vi "Instrument - Manual Object.vi"() -> ()   [LabVIEW 2020, in "Instrument Workspace Objects.lvlib"]
doc: "Sample numeric display item."
uses:
  Instrument Workspace Objects.lvlib
  <vilib>/NI VeriStand/Display Template Support/DisplayTemplateSupport.llb/cluster_Screen Item Settings.ctl
  <vilib>/NI VeriStand/Display Template Support/DisplayTemplateSupport.llb/cluster_Graph Scale Settings.ctl
  <vilib>/NI VeriStand/Display Template Support/DisplayTemplateSupport.llb/cluster_Graph Plot Settings.ctl
  NationalInstruments.VeriStand.SystemStorage
  Addon/Addon Shared/Types/Response Wait Type.ctl
  Workspace Shared/Types/State Variables.ctl
  <vilib>/NI VeriStand/Execution/Workspace/WorkspaceAPI.ctl
  <vilib>/NI VeriStand/Display Template Support/DisplayTemplateSupport.llb/enum_Display Template Handler Minimal To Workspace.ctl
  <vilib>/NI VeriStand/Display Template Support/DisplayTemplateSupport.llb/enum_Display Template Handler Minimal To Widget Msg.ctl
  <vilib>/NI/STM/TCP/TCP Connection Info.ctl
  <vilib>/NI/STM/SubVIs/MetaDataElement.ctl
  Workspace Shared/Types/CD Saved State.ctl
  <vilib>/NI VeriStand/Execution/Workspace/SystemStateEventRef.ctl
  <vilib>/NI VeriStand/Execution/Workspace/Target State Info.ctl
  <vilib>/NI VeriStand/Execution/Workspace/Target State.ctl
  <vilib>/NI VeriStand/Execution/Workspace/SystemStateRegEventRef.ctl
  Addon/Addon Shared/Types/Buffered RT Instrument Command.ctl
  <vilib>/NI VeriStand/Display Template Support/DisplayTemplateSupport.llb/sub_Display Template Handler Custom.vi
  Workspace Shared/Instrument Workspace Shared.lvlib
  <vilib>/NI VeriStand/Execution/Workspace/NI_VS Workspace ExecutionAPI.lvlib
  <vilib>/NI/STM/NI STM.lvlib
  APIs/Host Automation API/Instrument Host Automation API.lvlib
  Addon/Addon Shared/Instrument Addon Shared.lvlib
  NationalInstruments.VeriStand.ClientAPI
panel:
  in  "Command":string
  in  "Response?":bool
  in  "Wait Type":T1
  in  "Wait Value":dbl=100.0 format="%#_p"
  out "Timed Out?":bool
  out "Error Report":errorcluster
  out "Response":string
  in  "Send":bool
  out "Device":string
  in  "NIVS.Gateway IP Address":string
  in  "NIVS.System Definition Root":refnum<k24>
  in  "Item.Data":T2
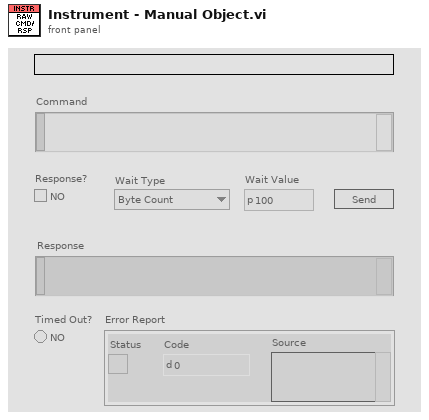
[diagram p1: front panel]
types:
  T1 = typedef "Instrument Addon Shared.lvlib/Response Wait Type.ctl" = enum16{"Byte Count", "Wait sec"}
  T2 = typedef "cluster_Screen Item Settings.ctl" = cluster{"Template VI":string, "Position X":i32, "Position Y":i32, "Custom":string, "Show Title Bar":bool, "ID":i32, "Always On Top":bool, "Allow Resize":bool, "Allow Minimize":bool, "Allow Close":bool, "Size to Screen":bool, "Screen.ID":i32, "State":enum16{"Normal", "New"}, "Title":string, "Window Bounds":cluster{"[0]":i16, "[1]":i16, "[2]":i16, "[3]":i16}, "Channel Ref":u64, "Unit":string, "Default Units?":bool, "Flash Limit?":bool, "Color 1":u32, "Color 2":u32, "Color 3":u32, "Color 4":u32, "Bck Color":u32, "Fore Color":u32, "Limit 1":dbl, "Limit 2":dbl, "Limit 3":dbl, "Limit 4":dbl, "Limit Mode 1":i32, "Limit Mode 2":i32, "Limit Mode 3":i32, "Limit Mode 4":i32, "Scale Precision":i32, "Scale Min":dbl, "Scale Max":dbl, "Format":i32, "Precision":i32, "Background Type":i32, "IDs":i32[], "Units":string[], "Labels":string[], "Scale Factor":dbl, "Scale Offset":dbl, "YScale Index":u32[], "XScale":T3, "YScales":T3[], "Plots":T4[], "Update Period":dbl, "History Length":dbl, "My.Ref":refnum<vi>, "Is Control?":bool, "Channel Paths":string[], "Custom Data":variant}
  T3 = typedef "cluster_Graph Scale Settings.ctl" = cluster{"Format":u8, "Precision":u8, "Fit":u8, "Label":string, "Use Default Label":bool, "Label Visible":bool, "Min":dbl, "Max":dbl}
  T4 = typedef "cluster_Graph Plot Settings.ctl" = cluster{"Bar Style":u8, "Fill To":i16, "Fill/PtColor":u32, "Line Style":u8, "Line Width":u8, "Color":u32, "Interp":u8, "Point Style":u8}
  T5 = typedef "Instrument Workspace Shared.lvlib/State Variables.ctl" = cluster{"UI.Device":refnum<vi>, "NIVS.Workspace":T6, "NIVS.SysDefRoot":refnum<k24>, "NIVS.CachedDataRef":refnum<user-event>, "NIVS.LaunchRef":refnum<user-event>, "Addon.Comm.Info":T7, "NIVS.CachedData":T9, "NIVS.SystemStateRefs":T10, "NIVS.UserEventRefs":cluster{"WorkspaceEvent":refnum<event-registration>, "SystemChangeEventRef":T11, "LaunchRef":refnum<event-registration>}, "NIVS.Workspace Event":refnum<event-registration>, "Addon.Connected?":bool, "Mode.Tool?":bool}
  T6 = typedef "NI_VS Workspace ExecutionAPI.lvlib/WorkspaceAPI.ctl" = refnum<k24>
  T7 = typedef "NI STM.lvlib/TCP Connection Info.ctl" = cluster{"connection ID":refnum<k5>, "meta data":T8[]}
  T8 = typedef "NI STM.lvlib/MetaDataElement.ctl" = string
  T9 = typedef "Instrument Workspace Shared.lvlib/CD Saved State.ctl" = cluster{"CD Path":string, "CD IP":string}
  T10 = typedef "NI_VS Workspace ExecutionAPI.lvlib/SystemStateEventRef.ctl" = cluster{"CustDatRef":refnum<user-event>, "EvtRef":refnum<k27>, "Target State User Event":refnum<user-event>}
  T11 = typedef "NI_VS Workspace ExecutionAPI.lvlib/SystemStateRegEventRef.ctl" = refnum<event-registration>
  T12 = typedef "enum_Display Template Handler Minimal To Workspace.ctl" = cluster{"Operation":enum16{"SetCustomData", "DeleteItem"}, "Data":variant}
  T13 = typedef "enum_Display Template Handler Minimal To Widget Msg.ctl" = enum16{"Stop", "LaunchConfigDialog"}
  T14 = typedef "Instrument Addon Shared.lvlib/Buffered RT Instrument Command.ctl" = cluster{"Command":string, "Response Expected?":bool, "Wait Type":T1, "Wait Value":dbl}
  T15 = enum8{"Enabled", "Disabled", "Disabled and Grayed Out"}
  T16 = cluster{"WorkspaceEvent":refnum<event-registration>, "SystemChangeEventRef":T11, "LaunchRef":refnum<event-registration>}
  T17 = typedef "Instrument Addon Shared.lvlib/Buffered RT Instrument Request.ctl" = cluster{"Response":string, "Error":errorcluster}
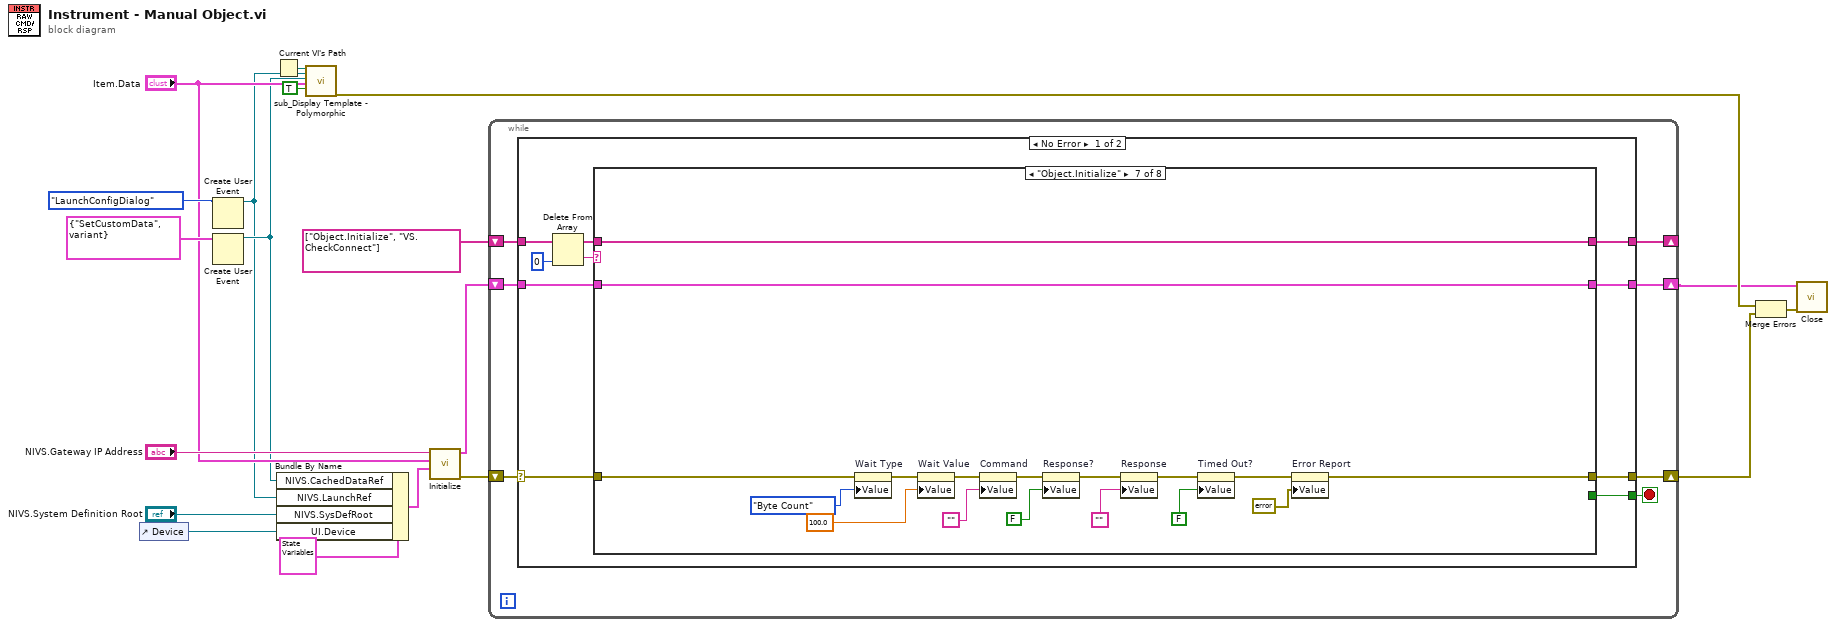
[diagram p0: block diagram]
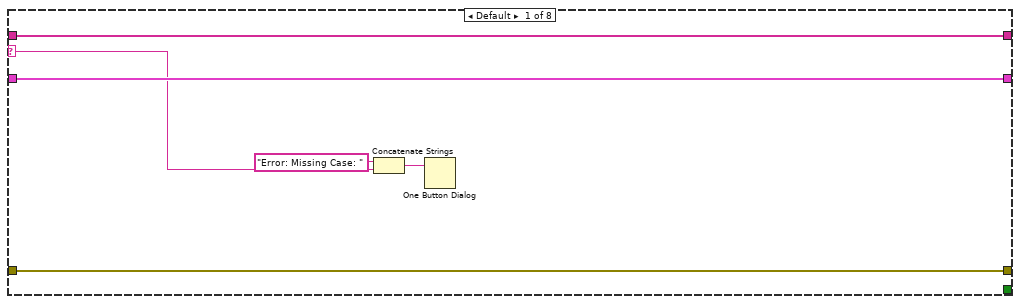
[diagram p2: hidden frame]
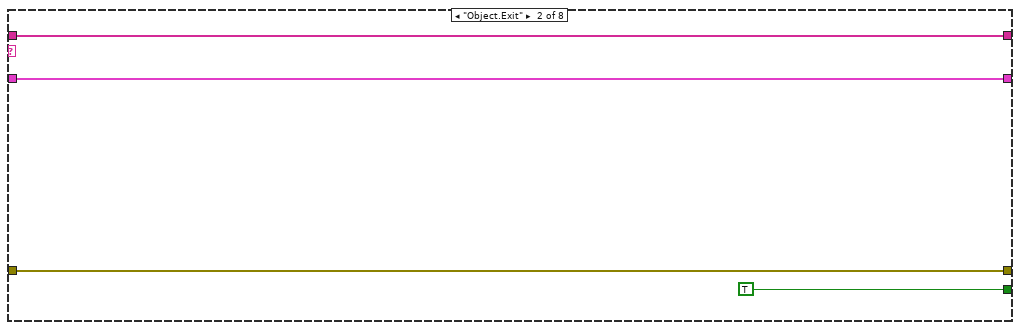
[diagram p3: hidden frame]
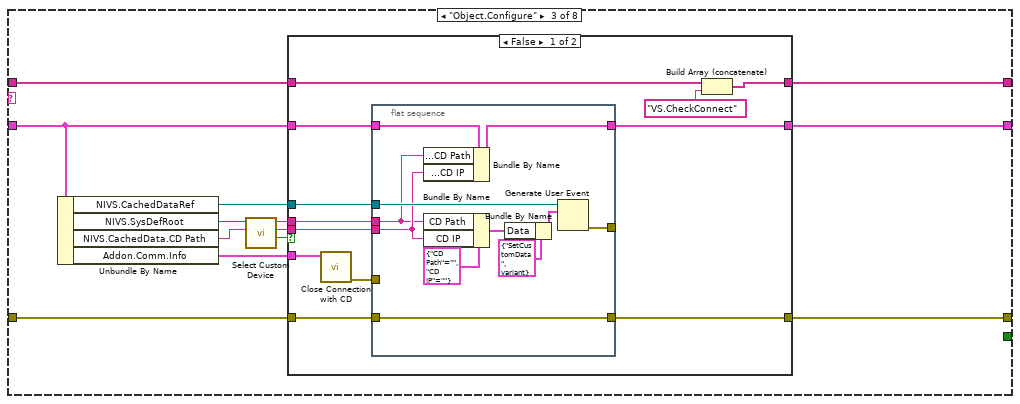
[diagram p4: hidden frame]
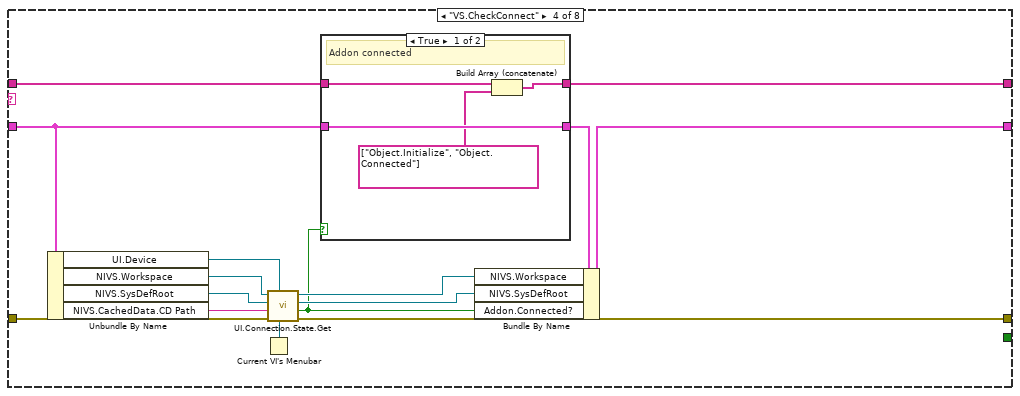
[diagram p6: hidden frame]
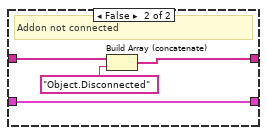
[diagram p7: hidden frame]
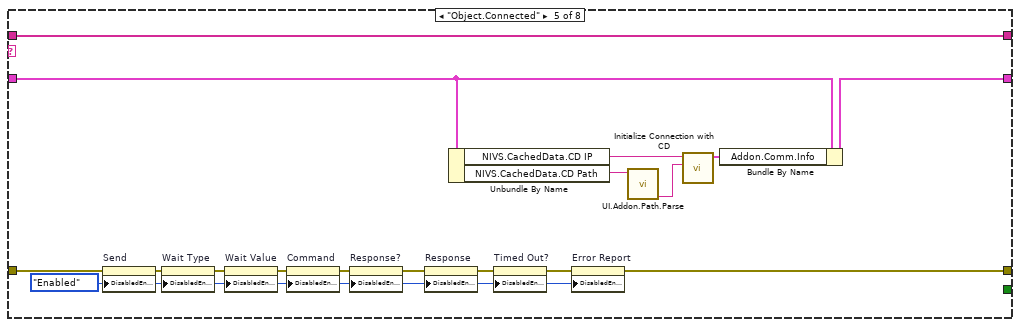
[diagram p8: hidden frame]
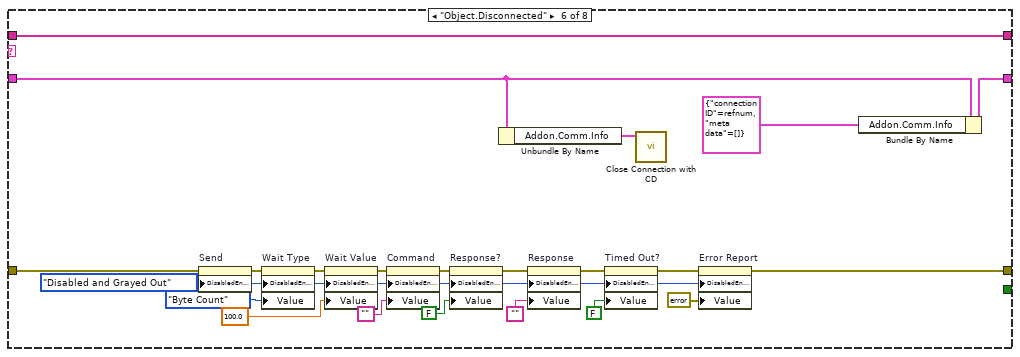
[diagram p9: hidden frame]
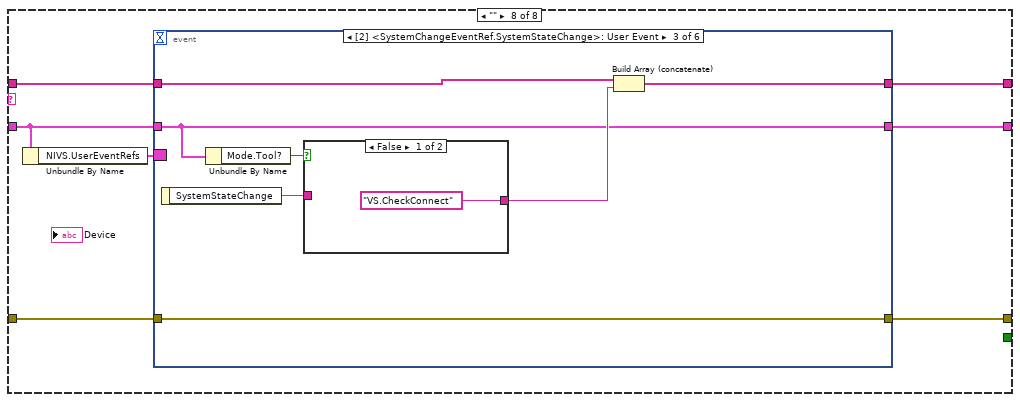
[diagram p10: hidden frame]
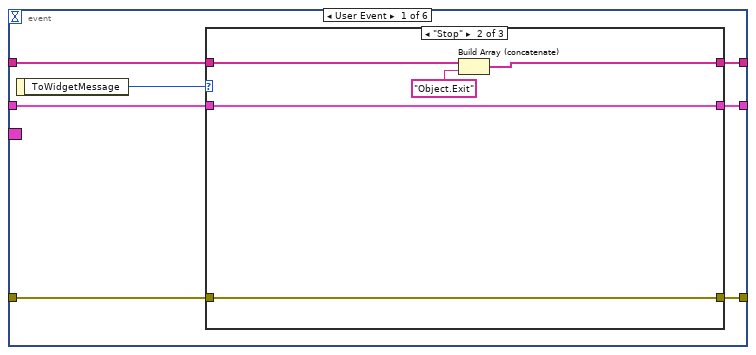
[diagram p11: hidden frame]
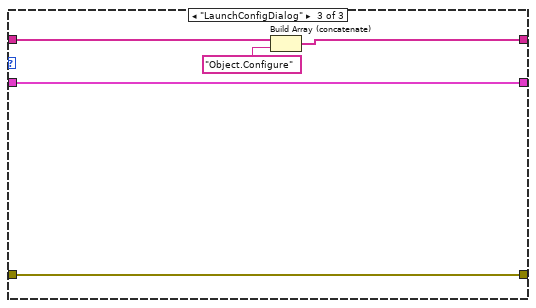
[diagram p13: hidden frame]
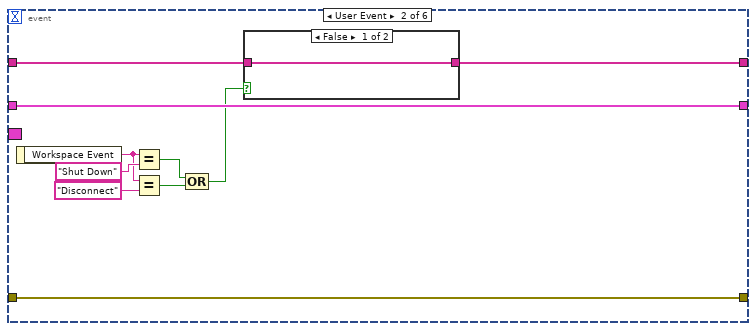
[diagram p14: hidden frame]
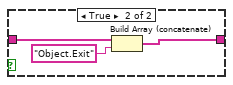
[diagram p15: hidden frame]
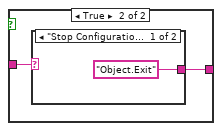
[diagram p16: hidden frame]
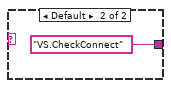
[diagram p17: hidden frame]
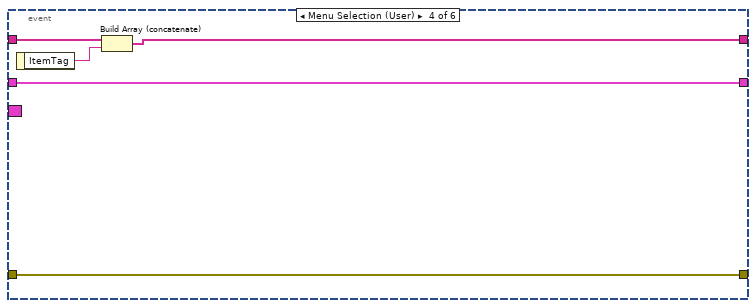
[diagram p18: hidden frame]
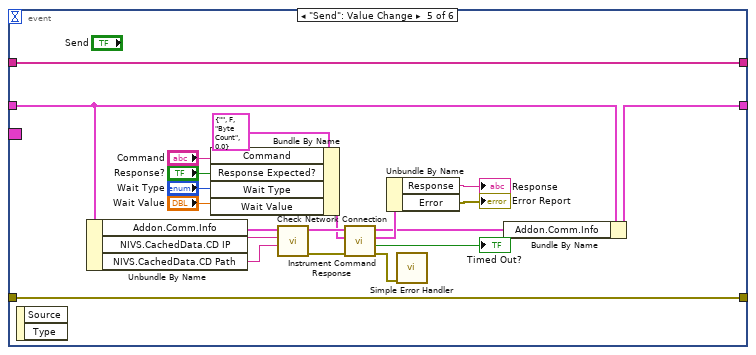
[diagram p19: hidden frame]
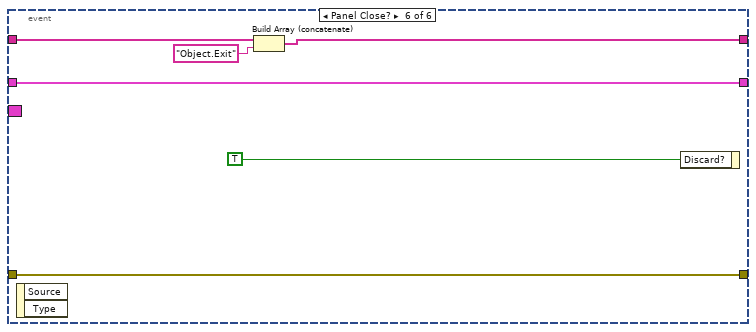
[diagram p20: hidden frame]
diagram:
  n1 = control-ref of="Device"() -> (w2:refnum<vi>)
  n2 = Create User Event(user event datatype=enum_Display_Template_Handler_Minimal_To_Widget_Msg."LaunchConfigDialog" ("ToWidgetMessage")) -> (user event=w9:refnum<user-event>)  [unwired: 1 in, 1 out]
  n3 = Create User Event(user event datatype=T12 {"Operation"=enum."SetCustomData", "Data"=variant} ("Data")) -> (user event=w10:refnum<user-event>)  [unwired: 1 in, 1 out]
  n4 = Current VI's Path() -> (path=w17:path)
  n5 = Bundle By Name(cluster=T5 {"UI.Device"=refnum, "NIVS.Workspace"=refnum, "NIVS.SysDefRoot"=refnum, "NIVS.CachedDataRef"=refnum, "NIVS.LaunchRef"=refnum, "Addon.Comm.Info"={"connection ID"=refnum, "meta data"=[]}, "NIVS.CachedData"={"CD Path"="", "CD IP"=""}, "NIVS.SystemStateRefs"={"CustDatRef"=refnum, "EvtRef"=refnum, "Target State User Event"=refnum}, "NIVS.UserEventRefs"={"WorkspaceEvent"=refnum, "SystemChangeEventRef"=refnum, "LaunchRef"=refnum}, "NIVS.Workspace Event"=refnum, "Addon.Connected?"=FALSE, "Mode.Tool?"=FALSE} ("State Variables in"), "NIVS.CachedDataRef"=w10, "NIVS.LaunchRef"=w9, "NIVS.SysDefRoot"="NIVS.System Definition Root", "UI.Device"=w2) -> (w11:T5)
  n6 = call-poly <vilib>:"sub_Display Template - Polymorphic.vi"("Parent.Path"=w17, "ToWidgetEvent"=w9, "ToWorkspace"=w10, "Item.Data"="Item.Data", "Resizable"=TRUE) -> ("error out"=w8:errorcluster)  [unwired: 1 in, 13 out]
  n7 = call "Initialize.vi"("State Variables in"=w11, "Item.Data"="Item.Data", "NIVS.Gateway IP Address"="NIVS.Gateway IP Address") -> ("error out"=w4:errorcluster, "State Variables out"=w5:T5)  [unwired: 7 in]
  n8 = while {
    shift-right: [w25] -> w1
    shift-left: w4 -> [w22]
    shift-right: [w23] -> w3
    shift-left: w5 -> [w24]
    shift-right: [w20] -> _
    shift-left: string[] ["Object.Initialize", "VS.CheckConnect"] -> [w21]
    stop <- w26 stop-if-true
    n9 = case shown="No Error" w22 {
      selector: w22 -> [w32 w251]
      tunnel: [w36 _] -> w26
      tunnel: [w35 w250] -> w25
      tunnel: w24 -> [w34 w254]
      tunnel: [w33 w254] -> w23
      tunnel: w21 -> [w30 w253]
      tunnel: [w27 w253] -> w20
      frame No Error {
        n10 = Delete From Array(array=w30, index=0) -> (deleted portion=w29:string, array with subset deleted=w28:string[])  [unwired: 1 in]
        n11 = case shown="\"Object.Initialize\"" w29 {
          selector: w29 -> [w39 _ _ _ _ _ _ _]
          tunnel: [_ TRUE _ _ _ _ _ _] -> w36
          tunnel: [w41 w45 w53 w90 w111 w131 w153 w171] -> w35
          tunnel: w34 -> [w42 w46 w54 w99 w121 w145 w148 w169]
          tunnel: [w42 w46 w52 w98 w120 w144 w148 w168] -> w33
          tunnel: w32 -> [w41 w45 w55 w91 w125 w126 w149 w167]
          tunnel: w28 -> [w40 w44 w48 w97 w124 w147 w164 w165]
          tunnel: [w40 w44 w47 w96 w124 w147 w164 w166] -> w27
          frame Default {
            n12 = Concatenate Strings("Error: Missing Case: " ("string"), w39) -> (w38:string)
            n13 = One Button Dialog(message=w38) -> ()  [unwired: 1 in, 1 out]
          }
          frame "Object.Exit" {
          }
          frame "Object.Configure" {
            n14 = Unbundle By Name(w54) -> ("NIVS.CachedDataRef"=w58:refnum<user-event>, "NIVS.SysDefRoot"=w59:refnum<k24>, "NIVS.CachedData.CD Path"=w56:string, "Addon.Comm.Info"=w57:T7)
            n15 = call "Select Custom Device.vi"("CD Path"=w56, "NIVS.System Definition Root"=w59) -> ("Cancelled?"=w51:bool, "IP Address"=w50:string, "Cached Addon Path"=w49:string)  [unwired: 7 in]
            n16 = case shown="False" w51 {
              tunnel: w58 -> [w71 _]
              tunnel: w50 -> [w69 _]
              tunnel: w49 -> [w70 _]
              tunnel: w57 -> [w68 _]
              tunnel: [w66 w85] -> w52
              tunnel: w54 -> [w65 w85]
              tunnel: [w63 w84] -> w53
              tunnel: w55 -> [w64 w84]
              tunnel: w48 -> [w62 w83]
              tunnel: [w60 w83] -> w47
              frame False {
                n17 = call "Close Connection with CD.vi"("Comm.Info"=w68) -> ("error out"=w67:errorcluster)  [unwired: 10 in]
                n18 = flat-sequence {
                  tunnel: w71 -> [w82]
                  tunnel: w70 -> [w73]
                  tunnel: w69 -> [w76]
                  tunnel: w67 -> [_]
                  tunnel: [w78] -> w66
                  tunnel: w65 -> [w79]
                  tunnel: [w74] -> _
                  tunnel: w64 -> [w72]
                  tunnel: [w72] -> w63
                  frame #0 {
                    n19 = Bundle By Name(cluster=w79, "NIVS.CachedData.CD Path"=w73, "NIVS.CachedData.CD IP"=w76) -> (w78:T5)
                    n20 = Bundle By Name(cluster=T9 {"CD Path"="", "CD IP"=""}, "CD Path"=w73, "CD IP"=w76) -> (w75:T9)
                    n21 = Bundle By Name(cluster=T12 {"Operation"=enum."SetCustomData", "Data"=variant} ("event data"), "Data"=w75) -> (w80:T12)
                    n22 = Generate User Event(user event=w82, event data cluster=w80) -> (error out=w74:errorcluster)  [unwired: 2 in, 1 out]
                  }
                }
                n23 = Build Array (concatenate)(w62, "VS.CheckConnect") -> (w60:string[])
              }
              frame True {
              }
            }
          }
          frame "VS.CheckConnect" {
            n24 = Unbundle By Name(w99) -> ("UI.Device"=w93:refnum<vi>, "NIVS.Workspace"=w95:T6, "NIVS.SysDefRoot"=w94:refnum<k24>, "NIVS.CachedData.CD Path"=w92:string)
            n25 = Current VI's Menubar() -> (w86:refnum<k9>)
            n26 = call "UI.Connection.State.Get.vi"("Menu Ref"=w86, "Name Ref"=w93, "error in (no error)"=w91, "Addon Path in"=w92, "NIVS.System Definition Root in"=w94, "NIVS.Workspace Ref in"=w95) -> ("error out"=w90:errorcluster, "Addon Connected?"=w87:bool, "NIVS.System Definition Root out"=w88:refnum<k24>, "NIVS.Workspace Ref out"=w89:T6)  [unwired: 2 in]
            n27 = case shown="True" w87 {
              tunnel: [w104 w108] -> w96
              tunnel: [w103 w106] -> w100
              tunnel: w99 -> [w103 w106]
              tunnel: w97 -> [w102 w105]
              frame True {
                # "Addon connected"
                n28 = Build Array (concatenate)(w102, string[] ["Object.Initialize", "Object.Connected"]) -> (w104:string[])
              }
              frame False {
                # "Addon not connected"
                n29 = Build Array (concatenate)(w105, "Object.Disconnected") -> (w108:string[])
              }
            }
            n30 = Bundle By Name(cluster=w100, "NIVS.Workspace"=w89, "NIVS.SysDefRoot"=w88, "Addon.Connected?"=w87) -> (w98:T5)
          }
          frame "Object.Connected" {
            w112 = T15."Enabled" ("Disabled")
            n31 = property on="Send" class="Bool"(error in=w125, "DisabledEnum"=w112) -> (error out=w116:errorcluster)  [unwired: 1 in, 1 out]
            n32 = property on="Wait Type" class="Enum (strict)"(error in=w116, "DisabledEnum"=w112) -> (error out=w119:errorcluster)  [unwired: 1 in, 1 out]
            n33 = property on="Wait Value" class="DigNum (strict)"(error in=w119, "DisabledEnum"=w112) -> (error out=w118:errorcluster)  [unwired: 1 in, 1 out]
            n34 = property on="Command" class="Str"(error in=w118, "DisabledEnum"=w112) -> (error out=w117:errorcluster)  [unwired: 1 in, 1 out]
            n35 = property on="Response?" class="Bool (strict)"(error in=w117, "DisabledEnum"=w112) -> (error out=w113:errorcluster)  [unwired: 1 in, 1 out]
            n36 = property on="Response" class="Str"(error in=w113, "DisabledEnum"=w112) -> (error out=w114:errorcluster)  [unwired: 1 in, 1 out]
            n37 = Unbundle By Name(w121) -> ("NIVS.CachedData.CD IP"=w123:string, "NIVS.CachedData.CD Path"=w110:string)
            n38 = property on="Timed Out?" class="Bool (strict)"(error in=w114, "DisabledEnum"=w112) -> (error out=w115:errorcluster)  [unwired: 1 in, 1 out]
            n39 = property on="Error Report" class="Clust (strict)"(error in=w115, "DisabledEnum"=w112) -> (error out=w111:errorcluster)  [unwired: 1 in, 1 out]
            n40 = call "UI.Addon.Path.Parse.vi"("Cached Addon Path"=w110) -> ("Addon Name"=w109:string)  [unwired: 6 in, 4 out]
            n41 = call "Initialize Connection with CD.vi"("TCP Service"=w109, "IP Address"=w123) -> ("connection info out"=w122:T7)  [unwired: 8 in, 1 out]
            n42 = Bundle By Name(cluster=w121, "Addon.Comm.Info"=w122) -> (w120:T5)
          }
          frame "Object.Disconnected" {
            w130 = T15."Disabled and Grayed Out" ("Disabled")
            n43 = property on="Send" class="Bool"(error in=w126, "DisabledEnum"=w130) -> (error out=w140:errorcluster)  [unwired: 1 in, 1 out]
            n44 = property on="Wait Type" class="Enum (strict)"(error in=w140, "DisabledEnum"=w130, "Value"=Response_Wait_Type."Byte Count" ("Wait Type")) -> (error out=w143:errorcluster)  [unwired: 1 in, 1 out]
            n45 = property on="Wait Value" class="DigNum (strict)"(error in=w143, "DisabledEnum"=w130, "Value"=100.0 ("Wait Value")) -> (error out=w142:errorcluster)  [unwired: 1 in, 1 out]
            n46 = property on="Command" class="Str"(error in=w142, "DisabledEnum"=w130, "Value"="") -> (error out=w141:errorcluster)  [unwired: 1 in, 1 out]
            n47 = property on="Response?" class="Bool (strict)"(error in=w141, "DisabledEnum"=w130, "Value"=FALSE ("Response?")) -> (error out=w132:errorcluster)  [unwired: 1 in, 1 out]
            n48 = Unbundle By Name(w145) -> ("Addon.Comm.Info"=w146:T7)
            n49 = property on="Response" class="Str"(error in=w132, "DisabledEnum"=w130, "Value"="") -> (error out=w133:errorcluster)  [unwired: 1 in, 1 out]
            n50 = property on="Timed Out?" class="Bool (strict)"(error in=w133, "DisabledEnum"=w130, "Value"=FALSE ("Response?")) -> (error out=w134:errorcluster)  [unwired: 1 in, 1 out]
            n51 = call "Close Connection with CD.vi"("Comm.Info"=w146) -> ()  [unwired: 10 in, 1 out]
            n52 = property on="Error Report" class="Clust (strict)"(error in=w134, "DisabledEnum"=w130, "Value"=errorcluster {"Status"=FALSE, "Code"=0, "Source"=""} ("Error Report")) -> (error out=w131:errorcluster)  [unwired: 1 in, 1 out]
            n53 = Bundle By Name(cluster=w145, "Addon.Comm.Info"=T7 {"connection ID"=refnum, "meta data"=[]} ("connection info")) -> (w144:T5)
          }
          frame "Object.Initialize" {
            n54 = property on="Wait Type" class="Enum (strict)"(error in=w149, "Value"=Response_Wait_Type."Byte Count" ("Wait Type")) -> (error out=w163:errorcluster)  [unwired: 1 in, 1 out]
            n55 = property on="Wait Value" class="DigNum (strict)"(error in=w163, "Value"=100.0 ("Wait Value")) -> (error out=w162:errorcluster)  [unwired: 1 in, 1 out]
            n56 = property on="Command" class="Str"(error in=w162, "Value"="") -> (error out=w161:errorcluster)  [unwired: 1 in, 1 out]
            n57 = property on="Response?" class="Bool (strict)"(error in=w161, "Value"=FALSE ("Response?")) -> (error out=w154:errorcluster)  [unwired: 1 in, 1 out]
            n58 = property on="Response" class="Str"(error in=w154, "Value"="") -> (error out=w155:errorcluster)  [unwired: 1 in, 1 out]
            n59 = property on="Timed Out?" class="Bool (strict)"(error in=w155, "Value"=FALSE ("Response?")) -> (error out=w156:errorcluster)  [unwired: 1 in, 1 out]
            n60 = property on="Error Report" class="Clust (strict)"(error in=w156, "Value"=errorcluster {"Status"=FALSE, "Code"=0, "Source"=""} ("Error Report")) -> (error out=w153:errorcluster)  [unwired: 1 in, 1 out]
          }
          frame "" {
            n61 = Unbundle By Name(w169) -> ("NIVS.UserEventRefs"=w170:T16)
            n62 = event shown="[2] <SystemChangeEventRef.SystemStateChange>: User Event" {
              selector: w170 -> [_ _ _ _ _ _]
              dyn-events: _ -> [_ _ _ _ _ _]
              timeout: _ -> [_ _ _ _ _ _]
              tunnel: [w177 w197 w207 w219 w225 w249] -> w168
              tunnel: w167 -> [w174 w192 w210 w218 w224 w248]
              tunnel: [w175 w192 w210 w218 w224 w248] -> w171
              tunnel: w169 -> [w176 w197 w207 w219 w226 w249]
              tunnel: [w173 w195 w211 w220 w223 w246] -> w166
              tunnel: w165 -> [w172 w194 w212 w222 w223 w245]
              event User Event {
                n63 = event-data() -> ("ToWidgetMessage"=w178:T13)  [unwired: 1 out]
                n64 = case shown="\"Stop\"" w178 {
                  tunnel: [w181 w186 w191] -> w177
                  tunnel: w176 -> [w181 w186 w191]
                  tunnel: [w180 w185 w190] -> w175
                  tunnel: w174 -> [w180 w185 w190]
                  tunnel: [w179 w183 w189] -> w173
                  tunnel: w172 -> [w179 w182 w188]
                  frame Default {
                  }
                  frame "Stop" {
                    n65 = Build Array (concatenate)(w182, "Object.Exit") -> (w183:string[])
                  }
                  frame "LaunchConfigDialog" {
                    n66 = Build Array (concatenate)(w188, "Object.Configure") -> (w189:string[])
                  }
                }
              }
              event User Event {
                n67 = event-data() -> ("Workspace Event"=w193:string)  [unwired: 1 out]
                n68 = Equal?(x=w193, y="Shut Down") -> (x = y?=w198:bool)
                n69 = Equal?(x=w193, y="Disconnect") -> (x = y?=w199:bool)
                n70 = Compound Arithmetic op=OR(w198, w199) -> (w196:bool)
                n71 = case shown="False" w196 {
                  tunnel: [w202 w204] -> w195
                  tunnel: w194 -> [w202 w203]
                  frame False {
                  }
                  frame True {
                    n72 = Build Array (concatenate)(w203, "Object.Exit") -> (w204:string[])
                  }
                }
              }
              event User Event {
                n73 = event-data() -> ("SystemStateChange"=w208:string)  [unwired: 1 out]
                n74 = Unbundle By Name(w207) -> ("Mode.Tool?"=w206:bool)
                n75 = case shown="False" w206 {
                  tunnel: ["VS.CheckConnect" w215] -> w209
                  tunnel: w208 -> [_ w214]
                  frame False {
                  }
                  frame True {
                    n76 = case shown="\"Stop Configuration\"" w214 {
                      tunnel: ["Object.Exit" "VS.CheckConnect"] -> w215
                      frame "Stop Configuration" {
                      }
                      frame Default {
                      }
                    }
                  }
                }
                n77 = Build Array (concatenate)(w212, w209) -> (w211:string[])
              }
              event Menu Selection (User) {
                n78 = event-data() -> ("ItemTag"=w221:string)  [unwired: 1 out]
                n79 = Build Array (concatenate)(w222, w221) -> (w220:string[])
              }
              event "Send": Value Change {
                n80 = event-data() -> ()  [unwired: 3 out]
                n81 = Unbundle By Name(w226) -> ("Addon.Comm.Info"=w228:T7, "NIVS.CachedData.CD IP"=w243:string, "NIVS.CachedData.CD Path"=w242:string)
                n82 = Bundle By Name(cluster=T14 {"Command"="", "Response Expected?"=FALSE, "Wait Type"=enum."Byte Count", "Wait Value"=0.0} ("Command Parameters"), "Command"="Command", "Response Expected?"="Response?", "Wait Type"="Wait Type", "Wait Value"="Wait Value") -> (w235:T14)
                n83 = call "Check Network Connection.vi"("CD Path"=w242, "IP Address"=w243, "Comm.Info"=w228) -> ("error out"=w240:errorcluster, "Comm.Info"=w241:T7)  [unwired: 7 in]
                n84 = call "Instrument Command Response.vi"("error in (no error)"=w240, "Command Parameters"=w235, "Comm.Info"=w241) -> ("error out"=w230:errorcluster, "Timed Out?"=→"Timed Out?":bool, "Response"=w233:T17, "Comm.Info"=w227:T7)  [unwired: 5 in]
                n85 = Unbundle By Name(w233) -> ("Response"=→"Response":string, "Error"=→"Error Report":errorcluster)
                n86 = call <vilib>:"Simple Error Handler.vi"("error in (no error)"=w230) -> ()  [unwired: 4 in, 5 out]
                n87 = Bundle By Name(cluster=w226, "Addon.Comm.Info"=w227) -> (w225:T5)
              }
              event Panel Close? {
                n88 = event-data() -> ()  [unwired: 3 out]
                n89 = Build Array (concatenate)(w245, "Object.Exit") -> (w246:string[])
                n90 = event-data("Discard?"=TRUE) -> ()  [unwired: 1 in, 1 out]
              }
            }
          }
        }
      }
      frame Error {
        n91 = call <vilib>:"Simple Error Handler.vi"("error in (no error)"=w251) -> ("error out"=w252:errorcluster)  [unwired: 4 in, 4 out]
        n92 = call <vilib>:"Clear Errors.vi"("error in (no error)"=w252) -> ("error out"=w250:errorcluster)  [unwired: 5 in, 1 out]
      }
    }
  }
  n93 = Merge Errors(w8, w1) -> (w7:errorcluster)
  n94 = call "Close.vi"("error in (no error)"=w7, "State Variables in"=w3) -> ()  [unwired: 10 in]
